vi "Process.vi"(8 "error in":errorcluster, 11 "Inst.RP100":refnum<class "Inst.RP100.lvclass">) -> (0 "error out":errorcluster, 3 "Inst.RP100 out":refnum<class "Inst.RP100.lvclass">)   [LabVIEW 2019, in "Inst.RP100.lvlib" / "Inst.RP100.lvclass"]
doc: "---------------------------------------------------------------\nJKI State Machine Objects™\nhttp://jki.net/state-machine-objects/\nCopyright (C) 2005-2015, JKI <info@jki.net>\nALL RIGHTS RESERVED"
uses:
  Inst.RP100.lvclass
  C:/Program Files (x86)/National Instruments/LabVIEW 2019/vi.lib/JKI/JKI SMO/SMO/SMO.lvclass
  C:/Program Files (x86)/National Instruments/LabVIEW 2019/user.lib/LevyLab/Instrument Framework/Instrument/Instrument.lvclass
  Typedefs/PrivateEvents--Inst.RP100.MessageToProcess.ctl
  <userlib>/LevyLab/RemoteControl/RemoteControl/Typedefs/Message--Cluster.ctl
  <vilib>/JKI/JKI SMO/SMO/SMO.lvclass/SMO.ctl
  Inst.RP100.lvclass/Inst.RP100.ctl
  <vilib>/JKI/JKI SMO/SMO/Private/ReftoDVR--SMO.vi
  <userlib>/LevyLab/Instrument Framework/Instrument Types/Strain/Instrument.Strain.lvclass
  <vilib>/JKI/JKI SMO/SMO/SMO.lvclass
  <userlib>/LevyLab/Instrument Framework/Instrument/Instrument.lvclass
  <userlib>/LevyLab/RemoteControl/RemoteControl/RemoteControl.lvclass
  <userlib>/LevyLab/Debug/Debug.lvlib
panel:
  out "Status":string
  out "State History":string
  # "Inst.RP100"
  # "Inst.RP100"
  # "For instructions on how to use the JKI State Machine Objects, examples and video tutorials, visit:\nhttp://jki.net/state-machine-objects/\n\nJKI State Machine Objects™\nhttp://jki.net/state-machine-objects/\nCopyright (C) 2005-2015, JKI <info@jki.net>\nALL RIGHTS RESERVED"
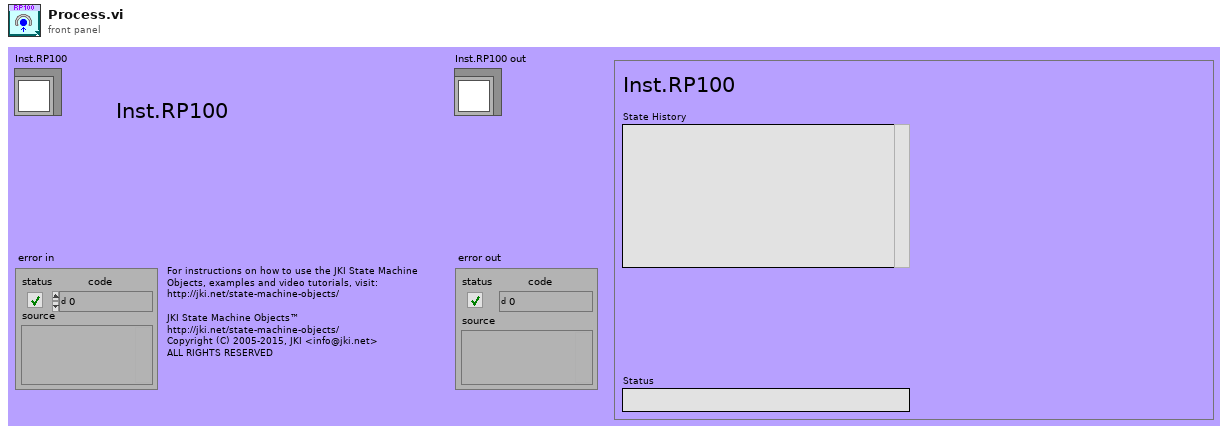
[diagram p1: front panel]
types:
  T1 = enum32{"invalid app kind", "Development System", "Run Time System", "Student Edition", "Embedded LabVIEW", "Evaluation", "Custom"}
  T2 = enum32{"Invalid", "Standard", "Closed", "Hidden", "Minimized", "Maximized"}
  T3 = typedef "RemoteControl.lvclass/Message--Cluster.ctl" = cluster{"Command":string, "Data":variant, "ID":string}
  T4 = typedef "Inst.RP100.lvlib/Inst.RP100.lvclass/PrivateEvents--Inst.RP100.MessageToProcess.ctl" = cluster{"Message":T5}
  T5 = typedef "RemoteControl.lvlib/RemoteControl.lvclass/Message--Cluster.ctl" = cluster{"Command":string, "Data":variant, "ID":string}
  T6 = cluster{"Core":cluster{"Current VI Reference":refnum<vi>, "Close Panel on Exit?":bool, "Last Error":cluster{"error":errorcluster, "previous state":string, "remaining states":string}, "Shutdown?":bool}, "SelfRef":refnum<class "Inst.RP100.lvclass">, "Running Step":i32, "sequence":string[], "MessageToProcess":T4}
  T7 = cluster{"Current VI Reference":refnum<vi>, "Close Panel on Exit?":bool, "Last Error":cluster{"error":errorcluster, "previous state":string, "remaining states":string}, "Shutdown?":bool}
  T8 = typedef "Debug.lvlib/Attribute.Debug.lvclass/DebugBehavior.ctl" = enum16{"Normal", "Debug"}
  T9 = typedef "smo.lvlib/SMO.lvclass/Protected Events.ctl" = cluster{"StopProcesses":refnum<user-event>, "AbortProcesses":refnum<user-event>, "Config Changed":refnum<user-event>, "Dependency":refnum<user-event>}
  T10 = typedef "Inst.RP100.lvlib/Inst.RP100.lvclass/Inst.RP100.getAll--Cluster.ctl" = cluster{"OutputStateCh1":string, "OutputStateCh2":string, "LevelCh1":dbl, "LevelCh2":dbl, "SlewCh1":dbl, "SlewCh2":dbl, "MeasuredVCh1":dbl, "MeasuredVCh2":dbl, "MeasuredICh1":dbl, "MeasuredICh2":dbl}
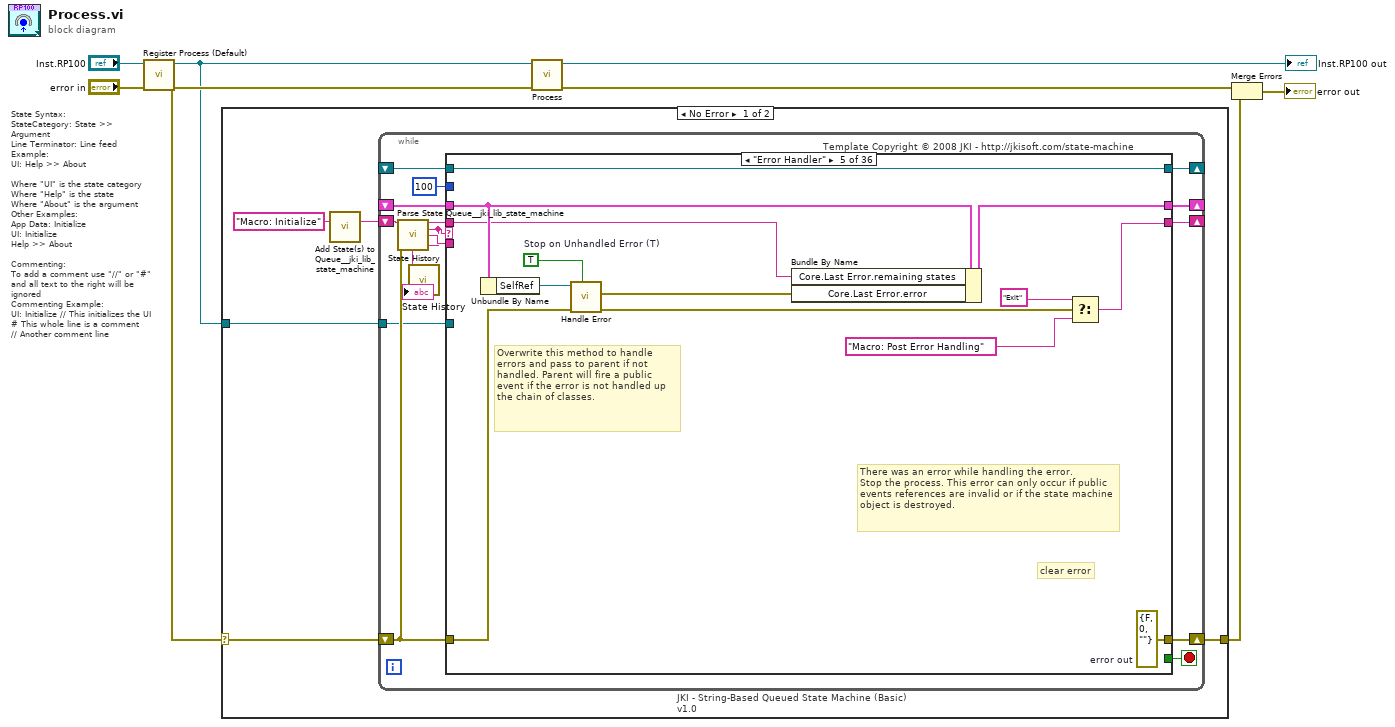
[diagram p0: block diagram]
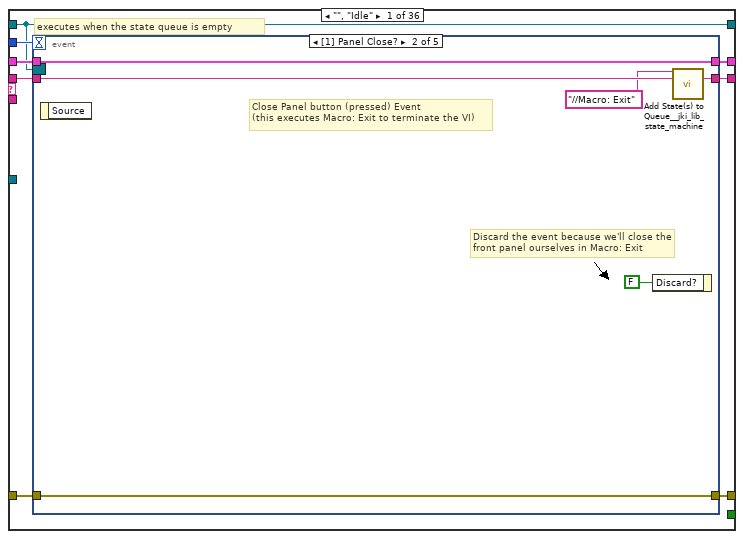
[diagram p2: hidden frame]
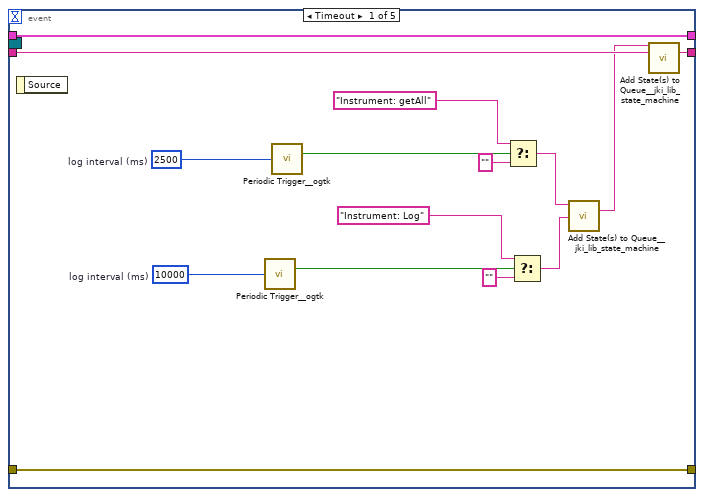
[diagram p3: hidden frame]
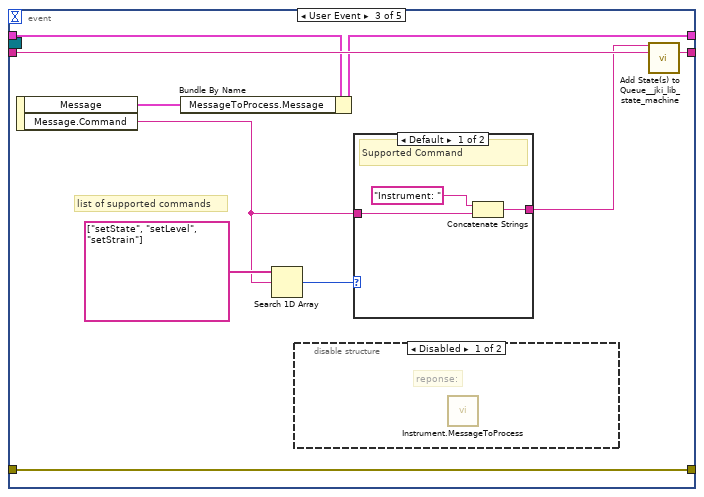
[diagram p4: hidden frame]
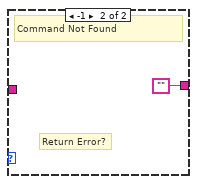
[diagram p6: hidden frame]
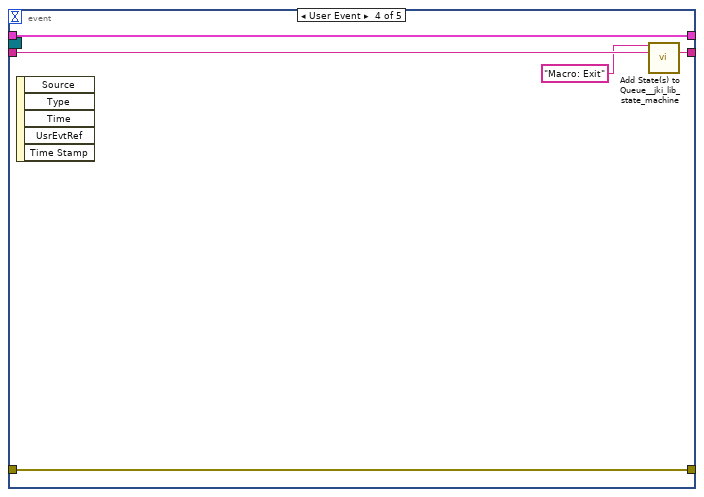
[diagram p7: hidden frame]
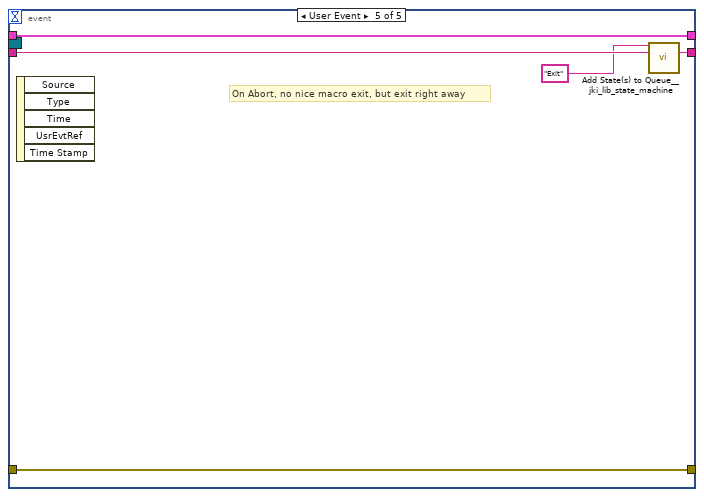
[diagram p8: hidden frame]
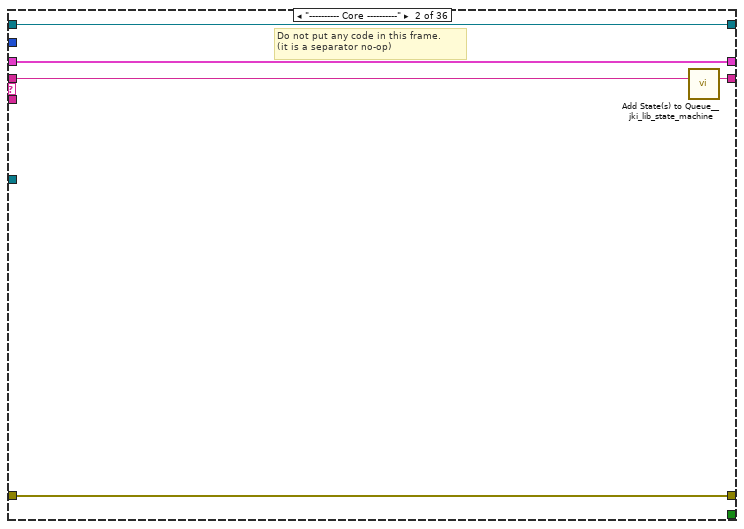
[diagram p9: hidden frame]
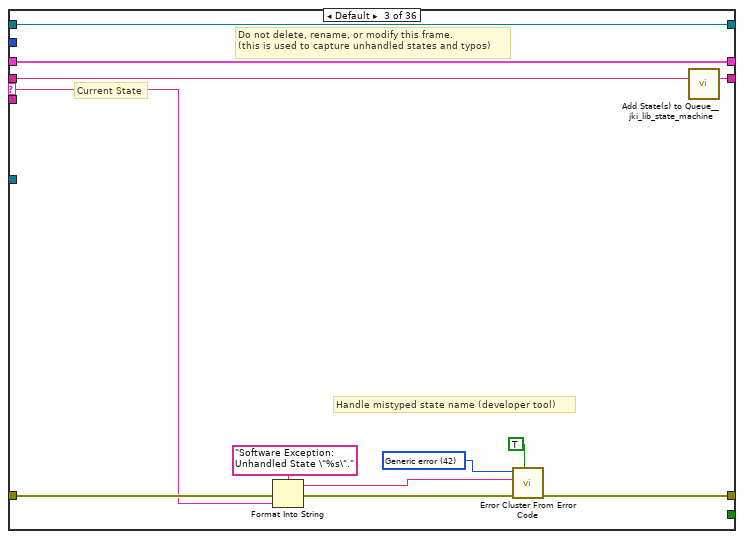
[diagram p10: hidden frame]
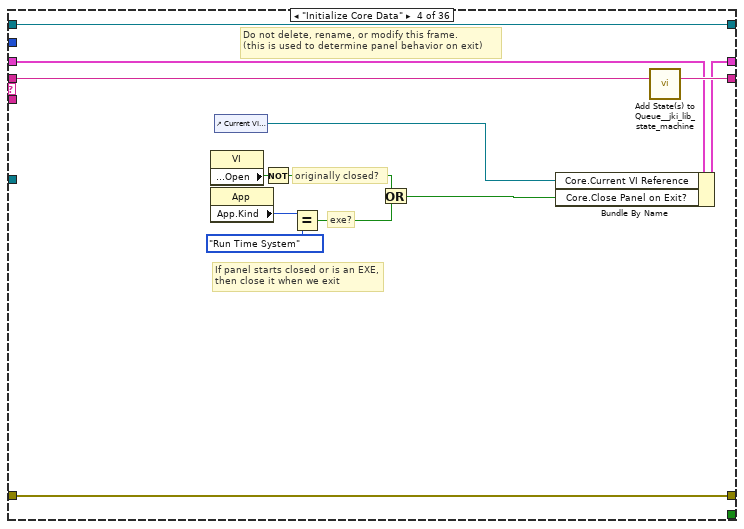
[diagram p11: hidden frame]
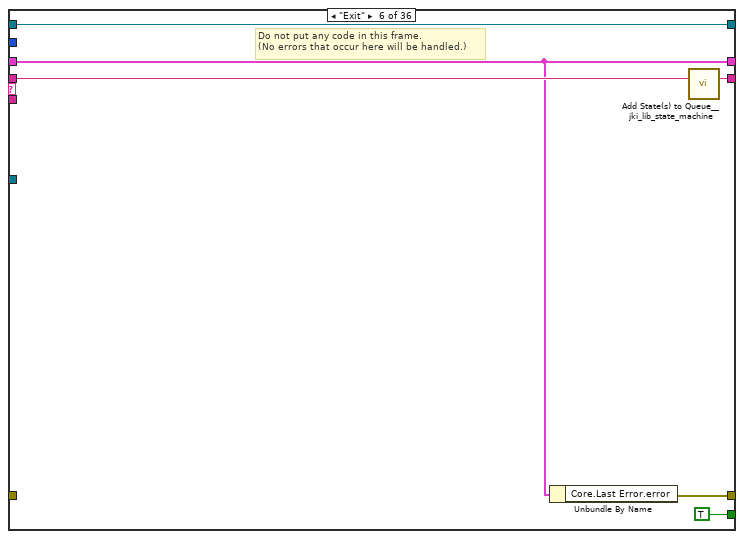
[diagram p12: hidden frame]
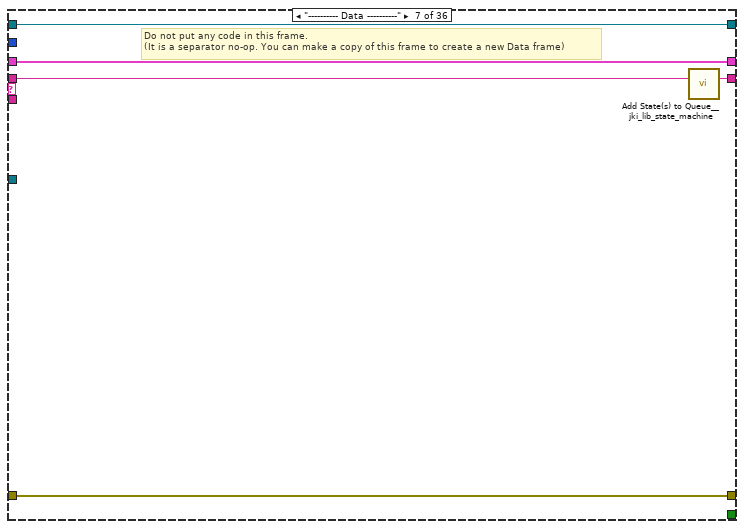
[diagram p13: hidden frame]
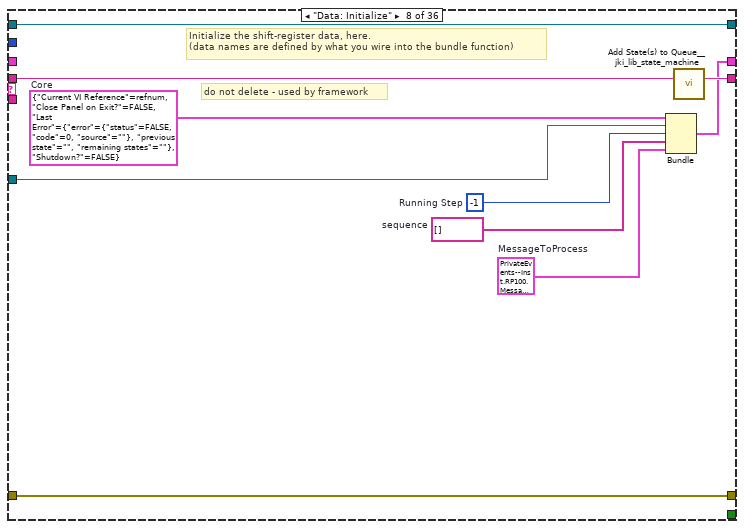
[diagram p14: hidden frame]
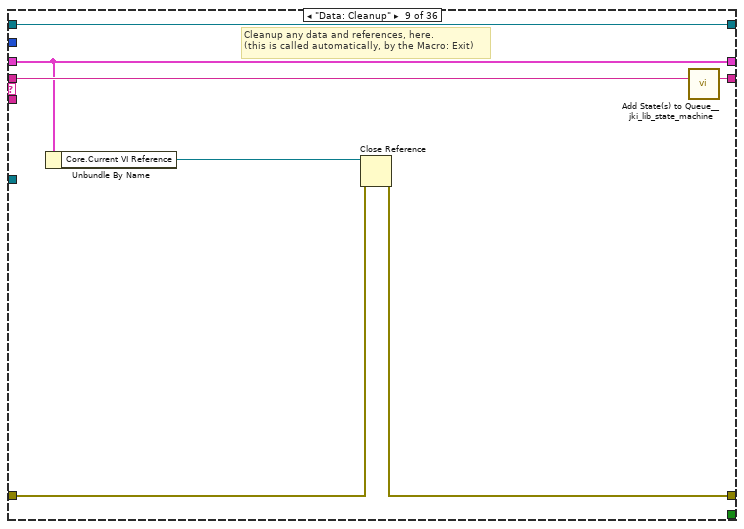
[diagram p15: hidden frame]
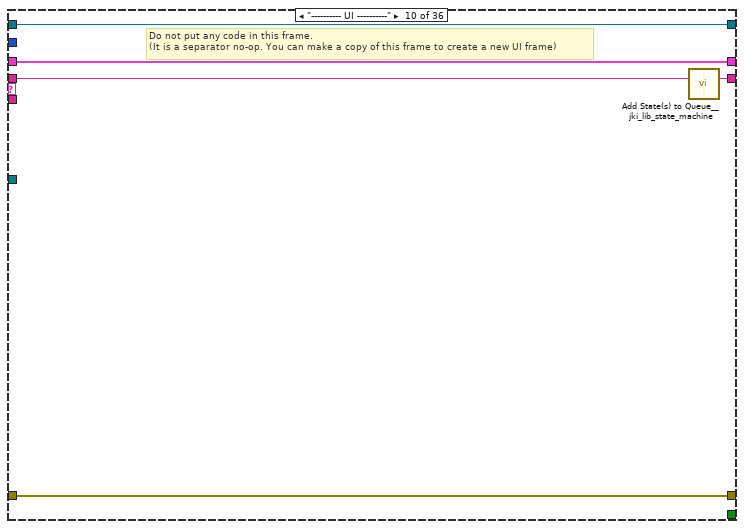
[diagram p16: hidden frame]
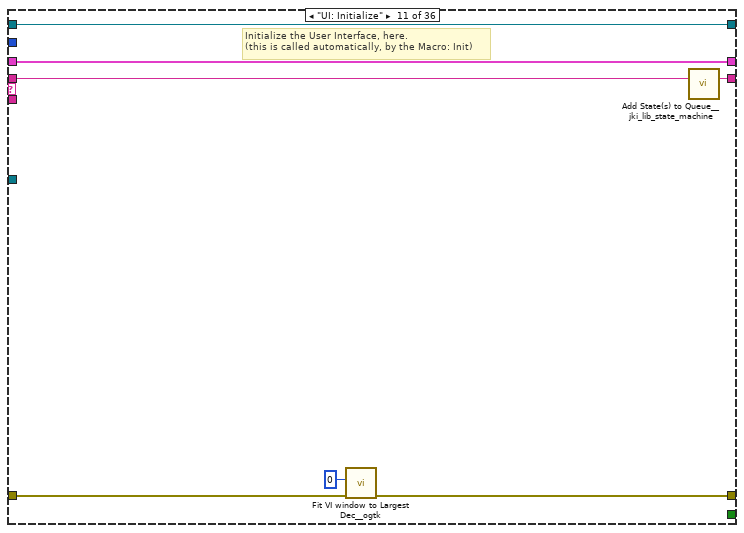
[diagram p17: hidden frame]
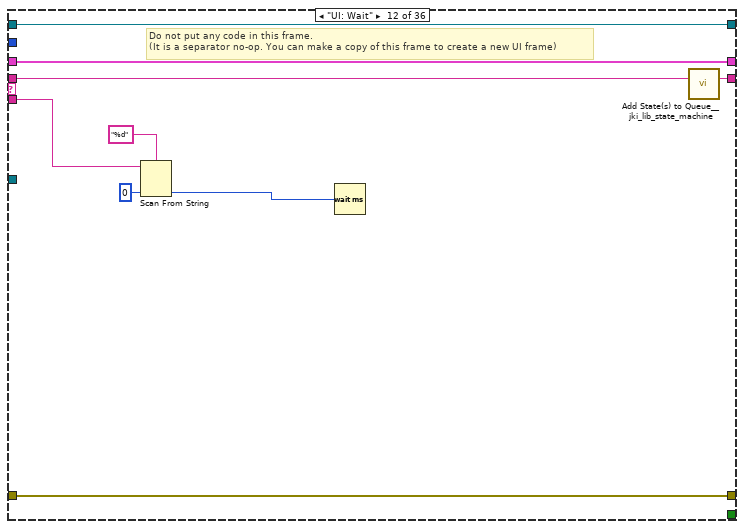
[diagram p18: hidden frame]
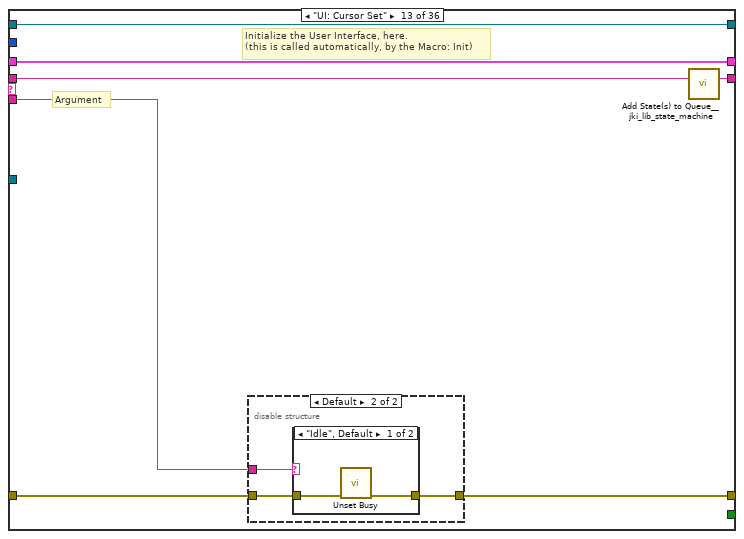
[diagram p19: hidden frame]
diagram:
  # "State Syntax:\nStateCategory: State >> Argument\nLine Terminator: Line feed\nExample:\nUI: Help >> About\n\nWhere \"UI\" is the state category\nWhere \"Help\" is the state\nWhere \"About\" is the argument\nOther Examples:\nApp Data: Initialize\nUI: Initialize\nHelp >> About\n\nCommenting:\nTo add a comment use \"//\" or \"#\" and all text to the right will be ignored\nCommenting Example:\nUI: Initialize // This initializes the UI\n# This whole line is a comment\n// Another comment line"
  n1 = call <vilib>:"Register Process (Default).vi"("error in (no error)"="error in", "SMO"="Inst.RP100") -> ("error out"=w5:errorcluster, "SelfRef"=w4:refnum<class "Inst.RP100.lvclass">)  [unwired: 8 in]
  n2 = case shown="No Error" w5 {
    selector: w5 -> [w10 w458]
    tunnel: w4 -> [w11 _]
    tunnel: [w9 w458] -> w1
    frame No Error {
      n3 = call <vilib>:"Add State(s) to Queue__jki_lib_state_machine.vi"("State(s) in (\"\")"="Macro: Initialize") -> ("States Out"=w13:string)  [unwired: 14 in]
      n4 = while "JKI - String-Based Queued State Machine (Basic) v1.0" {
        shift-right: [w22] -> _
        shift-left: _ -> [w21]
        shift-right: [w25] -> w9
        shift-left: w10 -> [w19]
        shift-right: [w24] -> _
        shift-left: w13 -> [w26]
        tunnel: w11 -> [w18]
        shift-right: [w17] -> _
        shift-left: _ -> [w16]
        stop <- w23 stop-if-true
        # "Template Copyright © 2008 JKI - http://jkisoft.com/state-machine"
        n5 = call <vilib>:"Parse State Queue__jki_lib_state_machine.vi"("State Queue"=w26, "Error In (no error)"=w19) -> ("Remaining States"=w28:string, "Current State"=w15:string, "Arguments"=w27:string)  [unwired: 11 in]
        n6 = call <userlib>:"State History.vi"("Current State"=w15) -> ("History"=→"State History":string)  [unwired: 10 in]
        n7 = case shown="\"Error Handler\"" w15 {
          selector: w15 -> [_ _ w88 _ _ _ _ _ _ _ _ _ _ _ _ _ _ _ _ _ _ _ _ _ _ _ _ _ _ _ _ _ _ _ _ _]
          tunnel: w28 -> [w36 w86 w92 w111 w116 w130 w135 w145 w152 w157 w164 w173 w180 w196 w228 w237 w252 w269 w290 w307 w312 w323 w328 w341 w347 w354 w363 w372 w382 w392 w402 w414 w427 w432 w438 w457]
          tunnel: w27 -> [_ _ _ _ _ _ _ _ _ _ _ w165 w174 w190 _ _ _ _ _ _ _ _ _ _ _ _ _ _ _ _ _ _ _ _ w433 w441]
          tunnel: w21 -> [w34 w83 w90 w102 w120 w126 w132 _ w146 w154 w162 w170 w178 w192 w225 w234 w241 w259 w280 w291 w309 w320 w325 w334 w345 w349 w359 w368 w378 w388 w398 w410 w423 w428 w434 w447]
          tunnel: [w33 w84 w94 w108 w121 w125 w133 w137 w148 w155 w159 w171 w175 w193 w226 w229 w239 w267 w288 w294 w310 w314 w326 w337 w343 w351 w356 w365 w374 w384 w394 w403 w417 w429 w435 w449] -> w25
          tunnel: w19 -> [w32 w84 w93 w108 w122 _ w133 w137 w149 w155 w158 w171 w176 w194 w226 w229 w238 w267 w288 w294 w310 w315 w326 w331 w343 w351 w355 w364 w375 w385 w395 w408 w418 w429 w435 w443]
          tunnel: [w35 w85 w91 w110 w112 w129 w134 w144 w151 w156 w163 w172 w179 w195 w227 w236 w251 w268 w289 w306 w311 w322 w327 w340 w346 w353 w362 w371 w381 w391 w401 w413 w426 w431 w437 w456] -> w24
          tunnel: [_ _ _ _ _ TRUE _ _ _ _ _ _ _ _ _ _ _ _ _ _ _ _ _ _ _ _ _ _ _ _ _ _ _ _ _ _] -> w23
          tunnel: [w31 w83 w90 w109 w119 w126 w132 w143 w146 w154 w162 w170 w178 w192 w225 w234 w242 w260 w281 w292 w309 w320 w325 w334 w345 w350 w360 w369 w379 w389 w399 w411 w424 w428 w434 w446] -> w22
          tunnel: 100 ("Timeout") -> [w30 _ _ _ _ _ _ _ _ _ _ _ _ _ _ _ _ _ _ _ _ _ _ _ _ _ _ _ _ _ _ _ _ _ _ _]
          tunnel: w18 -> [_ _ _ _ _ _ _ w138 _ _ _ _ _ _ _ _ _ _ _ _ _ _ _ _ _ _ _ _ _ _ _ _ _ _ _ _]
          tunnel: [w29 w82 w87 w99 w124 w127 w131 w142 w147 w153 w161 w169 w177 w189 w224 w235 w250 w266 w287 w301 w308 w321 w324 w339 w344 w352 w361 w370 w380 w390 w400 w412 w425 w430 w436 w455] -> w17
          tunnel: w16 -> [w29 w82 w87 w99 w124 w127 w131 w142 w147 w153 w161 w169 w177 w189 w224 w235 w250 w266 w287 w301 w308 w321 w324 _ w344 w352 w361 w370 w380 w390 w400 w412 w425 w430 w436 w455]
          frame "", "Idle" {
            # "executes when the state queue is empty"
            n8 = event shown="[1] Panel Close?" {
              selector: w29 -> [_ _ _ _ _]
              dyn-events: _ -> [_ _ _ _ _]
              timeout: w30 -> [_ _ _ _ _]
              tunnel: w36 -> [w51 w57 w67 w76 w81]
              tunnel: [w50 w56 w66 w75 w80] -> w35
              tunnel: w34 -> [w48 w54 w59 w73 w78]
              tunnel: [w49 w55 w65 w74 w79] -> w33
              tunnel: w32 -> [w49 w55 w65 w74 w79]
              tunnel: [w48 w54 w60 w73 w78] -> w31
              event Timeout {
                w41 = u32 10000  # log interval (ms)
                w45 = u32 2500  # log interval (ms)
                n9 = event-data() -> ()  [unwired: 1 in, 1 out]
                n10 = call <userlib>:"Periodic Trigger__ogtk.vi"("time (ms)"=w41) -> ("Triggered"=w40:bool)  [unwired: 12 in, 2 out]
                n11 = call <userlib>:"Periodic Trigger__ogtk.vi"("time (ms)"=w45) -> ("Triggered"=w47:bool)  [unwired: 12 in, 2 out]
                n12 = Select(t="Instrument: getAll", s=w47, f="") -> (s? t:f=w38:string)
                n13 = Select(t="Instrument: Log", s=w40, f="") -> (s? t:f=w39:string)
                n14 = call <vilib>:"Add State(s) to Queue__jki_lib_state_machine.vi"("State(s) in Front (\"\")"=w38, "State(s) at Back (\"\")"=w39) -> ("States Out"=w37:string)  [unwired: 13 in]
                n15 = call <vilib>:"Add State(s) to Queue__jki_lib_state_machine.vi"("State(s) in Front (\"\")"=w37, "State(s) in (\"\")"=w51) -> ("States Out"=w50:string)  [unwired: 13 in]
              }
              event Panel Close? {
                # "Discard the event because we'll close the front panel ourselves in Macro: Exit"
                # "Close Panel button (pressed) Event\n(this executes Macro: Exit to terminate the VI)"
                n16 = event-data() -> ()  [unwired: 1 in, 1 out]
                n17 = event-data("Discard?"=FALSE) -> ()  [unwired: 1 in, 1 out]
                n18 = call <vilib>:"Add State(s) to Queue__jki_lib_state_machine.vi"("State(s) in Front (\"\")"="//Macro: Exit", "State(s) in (\"\")"=w57) -> ("States Out"=w56:string)  [unwired: 13 in]
              }
              event User Event {
                # "list of supported commands"
                n19 = event-data() -> ("Message"=w58:T3, "Message.Command"=w61:string)  [unwired: 1 in]
                n20 = Bundle By Name(cluster=w59, "MessageToProcess.Message"=w58) -> (w60:T6)
                n21 = Search 1D Array(1D array=string[] ["setState", "setLevel", "setStrain"], element=w61) -> (index of element=w64:i32)  [unwired: 1 in]
                n22 = disable-structure shown="Disabled" {
                  frame Disabled {
                    # "reponse:"
                    n23 = call <userlib>:"Instrument.MessageToProcess.vi"() -> ()  [unwired: 10 in, 2 out]
                  }
                  frame Enabled {
                  }
                }
                n24 = case shown="Default" w64 {
                  tunnel: [w70 "" ("Empty String Constant")] -> w62
                  tunnel: w61 -> [w69 _]
                  frame Default {
                    # "Supported Command"
                    n25 = Concatenate Strings("Instrument: ", w69) -> (w70:string)
                  }
                  frame -1 {
                    # "Return Error?"
                    # "Command Not Found"
                  }
                }
                n26 = call <vilib>:"Add State(s) to Queue__jki_lib_state_machine.vi"("State(s) in Front (\"\")"=w62, "State(s) in (\"\")"=w67) -> ("States Out"=w66:string)  [unwired: 13 in]
              }
              event User Event {
                n27 = event-data() -> ()  [unwired: 1 in, 5 out]
                n28 = call <vilib>:"Add State(s) to Queue__jki_lib_state_machine.vi"("State(s) in Front (\"\")"="Macro: Exit", "State(s) in (\"\")"=w76) -> ("States Out"=w75:string)  [unwired: 13 in]
              }
              event User Event {
                # "On Abort, no nice macro exit, but exit right away"
                n29 = event-data() -> ()  [unwired: 1 in, 5 out]
                n30 = call <vilib>:"Add State(s) to Queue__jki_lib_state_machine.vi"("State(s) in Front (\"\")"="Exit", "State(s) in (\"\")"=w81) -> ("States Out"=w80:string)  [unwired: 13 in]
              }
            }
          }
          frame "---------- Core ----------" {
            # "Do not put any code in this frame.\n(it is a separator no-op)"
            n31 = call <vilib>:"Add State(s) to Queue__jki_lib_state_machine.vi"("State(s) in (\"\")"=w86) -> ("States Out"=w85:string)  [unwired: 14 in]
          }
          frame Default {
            w97 = 42 items=["No error", "Argument error", "Memory is full", "Out of zone", "End of file", "File already open", "Generic file I/O error", "File not found", "File permission error", "Disk is full", "Duplicate path", "Too many files open", "System feature not enabled", "Resource file not found", "Cannot add resource", "Resource not found", "Image not found", "Image memory error", "Pen does not exist", "Config type invalid", "Config token not found", "Config parse error", "Config memory error", "Bad external code format", "Bad external code offset", "External code not present", "Null window", "Destroy window error", "Null menu", "Print aborted", "Bad print record", "Print driver error", "Windows error during printing", "Memory error during printing", "Print dialog error", "Generic print error", "Invalid device refnum", "Device not found", "Device parameter error", "Device unit error", "Cannot open device", "Device call aborted", "Generic error", "Cancelled by user", "Object ID too low", "Object ID too high", "Object not in heap", "Unknown heap", "Unknown object (invalid DefProc)", "Unknown object (DefProc not in table)", "Message out of range", "Invalid (null) method", "Unknown message", "Manager call not supported", "Bad address", "Network operation in progress", "Network operation timed out", "Connection is busy", "Network attribute not supported", "Network error", "Address in use", "System out of memory", "Connection aborted", "Connection refused", "Not connected", "Already connected", "Connection closed", "Initialization error (interapplication manager)", "Bad occurrence", "Wait on unbound occurrence handler", "Occurrence queue overflow", "Datalog type conflict", "Unused", "Unrecognized type (interapplication manager)", "Memory corrupt", "Failed to make temporary DLL", "Old CIN version", "Drag socket not found", "Failed to load drop-object", "Failed to register OLE object", "Failed to release OLE object", "Format specifier type mismatch", "Unknown format specifier", "Too few format specifiers", "Too many format specifiers", "Scan failed", "Newer CIN version", "Error converting to variant", "Runtime menu error", "Password tampered", "Variant attribute not found", "Incompatible variant data type", "Event data is not available", "Event Store is not present", "Occurrence is not found", "Event Queue is not created", "Event info is not available", "Refnum passed is NULL", "Error retrieving Class GUID", "Error retrieving CoClass GUID", "Error retrieving TypeLib GUID.", "Bad built application magic bytes.", "Specific driver is different from the specific driver associated with the Logical Name.", "There is no session opened to the class driver.", "Max Error", "MAX - Error with config objects", "MAX - Error loading configuration", "MAX - Group not supported"]
            # "Current State"
            # "Do not delete, rename, or modify this frame.\n(this is used to capture unhandled states and typos)"
            # "Handle mistyped state name (developer tool)"
            n32 = Format Into String(format string="Software Exception: Unhandled State \"%s\"." ("message"), error in=w93, w88) -> (resulting string=w96:string, error out=w95:errorcluster)  [unwired: 1 in]
            n33 = call <vilib>:"Error Cluster From Error Code.vi"("show call chain? (False)"=TRUE, "error in (no error)"=w95, "error message (\"\")"=w96, "error code (0)"=w97) -> ("error out"=w94:errorcluster)  [unwired: 5 in]
            n34 = call <vilib>:"Add State(s) to Queue__jki_lib_state_machine.vi"("State(s) in (\"\")"=w92) -> ("States Out"=w91:string)  [unwired: 14 in]
          }
          frame "Initialize Core Data" {
            # "Do not delete, rename, or modify this frame.\n(this is used to determine panel behavior on exit)"
            # "originally closed?"
            # "exe?"
            # "If panel starts closed or is an EXE, then close it when we exit"
            n35 = property class="VI"() -> ("Front Panel.Open"=w107:bool)  [unwired: 2 in, 2 out]
            n36 = property class="App"() -> ("App.Kind"=w106:T1)  [unwired: 2 in, 2 out]
            n37 = control-ref of="Current VI Reference"() -> (w100:refnum<vi>)
            n38 = Not(x=w107) -> (.not. x?=w104:bool)
            n39 = Equal?(x=w106, y=T1."Run Time System" ("Application:Kind")) -> (x = y?=w103:bool)
            n40 = Or(x=w104, y=w103) -> (x .or. y?=w101:bool)
            n41 = Bundle By Name(cluster=w102, "Core.Current VI Reference"=w100, "Core.Close Panel on Exit?"=w101) -> (w109:T6)
            n42 = call <vilib>:"Add State(s) to Queue__jki_lib_state_machine.vi"("State(s) in (\"\")"=w111) -> ("States Out"=w110:string)  [unwired: 14 in]
          }
          frame "Error Handler" {
            w117 = TRUE  # Stop on Unhandled Error (T)
            w121 = errorcluster {"status"=FALSE, "code"=0, "source"=""}  # error out
            # "clear error"
            # "There was an error while handling the error.\nStop the process. This error can only occur if public events references are invalid or if the state machine object is destroyed."
            # "Overwrite this method to handle errors and pass to parent if not handled. Parent will fire a public event if the error is not handled up the chain of classes."
            n43 = Unbundle By Name(w120) -> ("SelfRef"=w123:refnum<class "Inst.RP100.lvclass">)
            n44 = call-dynamic "Handle Error.vi"("Stop on Unhandled Error (T)"=w117, "error in"=w122, "SMO"=w123) -> ("handling error"=w113:errorcluster, "Unhandled error"=w118:errorcluster)  [unwired: 6 in, 1 out]
            n45 = Bundle By Name(cluster=w120, "Core.Last Error.remaining states"=w116, "Core.Last Error.error"=w118) -> (w119:T6)
            n46 = Select(t="Exit", s=w113, f="Macro: Post Error Handling") -> (s? t:f=w112:string)
          }
          frame "Exit" {
            # "Do not put any code in this frame.\n(No errors that occur here will be handled.)"
            n47 = Unbundle By Name(w126) -> ("Core.Last Error.error"=w125:errorcluster)
            n48 = call <vilib>:"Add State(s) to Queue__jki_lib_state_machine.vi"("State(s) in (\"\")"=w130) -> ("States Out"=w129:string)  [unwired: 14 in]
          }
          frame "---------- Data ----------" {
            # "Do not put any code in this frame.\n(It is a separator no-op. You can make a copy of this frame to create a new Data frame)"
            n49 = call <vilib>:"Add State(s) to Queue__jki_lib_state_machine.vi"("State(s) in (\"\")"=w135) -> ("States Out"=w134:string)  [unwired: 14 in]
          }
          frame "Data: Initialize" {
            w136 = T4 {"Message"={"Command"="", "Data"=variant(string ""), "ID"=""}}  # MessageToProcess
            w139 = string[] []  # sequence
            w140 = -1  # Running Step
            w141 = T7 {"Current VI Reference"=refnum, "Close Panel on Exit?"=FALSE, "Last Error"={"error"={"status"=FALSE, "code"=0, "source"=""}, "previous state"="", "remaining states"=""}, "Shutdown?"=FALSE}  # Core
            # "do not delete - used by framework"
            # "Initialize the shift-register data, here.\n(data names are defined by what you wire into the bundle function)"
            n50 = Bundle("Core"=w141, "SelfRef"=w138, "Running Step"=w140, "sequence"=w139, "MessageToProcess"=w136) -> (w143:T6)  [unwired: 1 in]
            n51 = call <vilib>:"Add State(s) to Queue__jki_lib_state_machine.vi"("State(s) in (\"\")"=w145) -> ("States Out"=w144:string)  [unwired: 14 in]
          }
          frame "Data: Cleanup" {
            # "Cleanup any data and references, here.\n(this is called automatically, by the Macro: Exit)"
            n52 = Unbundle By Name(w146) -> ("Core.Current VI Reference"=w150:refnum<vi>)
            n53 = Close Reference(reference=w150, error in (no error)=w149) -> (error out=w148:errorcluster)
            n54 = call <vilib>:"Add State(s) to Queue__jki_lib_state_machine.vi"("State(s) in (\"\")"=w152) -> ("States Out"=w151:string)  [unwired: 14 in]
          }
          frame "---------- UI ----------" {
            # "Do not put any code in this frame.\n(It is a separator no-op. You can make a copy of this frame to create a new UI frame)"
            n55 = call <vilib>:"Add State(s) to Queue__jki_lib_state_machine.vi"("State(s) in (\"\")"=w157) -> ("States Out"=w156:string)  [unwired: 14 in]
          }
          frame "UI: Initialize" {
            # "Initialize the User Interface, here.\n(this is called automatically, by the Macro: Init)"
            n56 = call <userlib>:"Fit VI window to Largest Dec__ogtk.vi"("error in (no error)"=w158, "border spacing (2 px)"=0) -> ("error out"=w159:errorcluster)  [unwired: 4 in, 1 out]
            n57 = call <vilib>:"Add State(s) to Queue__jki_lib_state_machine.vi"("State(s) in (\"\")"=w164) -> ("States Out"=w163:string)  [unwired: 14 in]
          }
          frame "UI: Wait" {
            # "Do not put any code in this frame.\n(It is a separator no-op. You can make a copy of this frame to create a new UI frame)"
            n58 = Scan From String(format string="%d", input string=w165, default 1=u32 0 ("default value 1")) -> (output 1=w166:u32)  [unwired: 2 in, 3 out]
            n59 = Wait (ms)(milliseconds to wait=w166) -> ()  [unwired: 1 out]
            n60 = call <vilib>:"Add State(s) to Queue__jki_lib_state_machine.vi"("State(s) in (\"\")"=w173) -> ("States Out"=w172:string)  [unwired: 14 in]
          }
          frame "UI: Cursor Set" {
            # "Argument"
            # "Initialize the User Interface, here.\n(this is called automatically, by the Macro: Init)"
            n61 = disable-structure shown="Default" {
              disable-tunnel: w176 -> [w181 w184]
              disable-tunnel: [w181 w183] -> w175
              disable-tunnel: w174 -> [_ w182]
              frame condition #0 {
              }
              frame condition #1 (active) {
                n62 = case shown="\"Idle\", Default" w182 {
                  tunnel: w184 -> [w186 w188]
                  tunnel: [w185 w187] -> w183
                  frame "Idle", Default {
                    n63 = call <vilib>:"Unset Busy.vi"("error in (no error)"=w186) -> ("error out"=w185:errorcluster)  [unwired: 10 in]
                  }
                  frame "Busy" {
                    n64 = call <vilib>:"Set Busy.vi"("error in (no error)"=w188) -> ("error out"=w187:errorcluster)  [unwired: 9 in, 1 out]
                  }
                }
              }
            }
            n65 = call <vilib>:"Add State(s) to Queue__jki_lib_state_machine.vi"("State(s) in (\"\")"=w180) -> ("States Out"=w179:string)  [unwired: 14 in]
          }
          frame "UI: Front Panel State" {
            # "Argument"
            # "Set Front Panel Open or Closed\n(Usage: \"UI: Front Panel State >> Open|Close\")"
            n66 = Unbundle By Name(w192) -> ("Core.Current VI Reference"=w191:refnum<vi>)
            n67 = disable-structure shown="Default" {
              disable-tunnel: w194 -> [w200 w223]
              disable-tunnel: [w199 w223] -> w193
              disable-tunnel: w191 -> [w198 _]
              disable-tunnel: w190 -> [w197 _]
              frame condition #0 (active) {
                n68 = case shown="\"Close\"" w197 {
                  tunnel: w200 -> [w204 w217]
                  tunnel: [w206 w218] -> w199
                  tunnel: w198 -> [w205 w215]
                  frame "Open", Default {
                    n69 = property class="VI"(reference=w205, error in=w204) -> (reference out=w202:refnum<vi>, error out=w203:errorcluster, "FP.State"=w201:T2)
                    n70 = case shown="\"Closed\"" w201 {
                      tunnel: [w209 w212] -> w206
                      tunnel: w203 -> [w208 w212]
                      tunnel: w202 -> [w207 _]
                      frame "Closed" {
                        n71 = invoke class="VI" method="FP.Open"(reference=w207, error in=w208, "Activate"=TRUE, "State"=T2."Standard") -> (error out=w209:errorcluster)  [unwired: 1 in, 4 out]
                      }
                      frame Default {
                      }
                    }
                  }
                  frame "Close" {
                    n72 = property class="VI"(reference=w215, error in=w217) -> (reference out=w214:refnum<vi>, error out=w216:errorcluster, "FP.State"=w213:T2)
                    n73 = case shown="Default" w213 {
                      tunnel: [w219 w222] -> w218
                      tunnel: w216 -> [w219 w221]
                      tunnel: w214 -> [_ w220]
                      frame "Invalid", "Closed" {
                      }
                      frame Default {
                        n74 = invoke class="VI" method="FP.Close"(reference=w220, error in=w221) -> (error out=w222:errorcluster)  [unwired: 1 in, 2 out]
                      }
                    }
                  }
                }
              }
              frame condition #1 {
              }
            }
            n75 = call <vilib>:"Add State(s) to Queue__jki_lib_state_machine.vi"("State(s) in (\"\")"=w196) -> ("States Out"=w195:string)  [unwired: 14 in]
          }
          frame "---------- Macro ----------" {
            # "Do not put any code in this frame.\n(It is a separator no-op. You can make a copy of this frame to create a new Macro frame)"
            n76 = call <vilib>:"Add State(s) to Queue__jki_lib_state_machine.vi"("State(s) in (\"\")"=w228) -> ("States Out"=w227:string)  [unwired: 14 in]
          }
          frame "Macro: Initialize" {
            # "Initialization Macro\n(This is called once, when the VI starts)"
            n77 = call <vilib>:"Add State(s) to Queue__jki_lib_state_machine.vi"("State(s) in Front (\"\")"="Data: Initialize\nInitialize Core Data\nEvents: Register", "State(s) in (\"\")"="Process: Sync", "State(s) at Back (\"\")"="UI: Initialize\nUI: Front Panel State >> Close\nInstrument: Open Hardware\nMacro: Debug") -> ("States Out"=w232:string)  [unwired: 12 in]
            n78 = call <vilib>:"Add State(s) to Queue__jki_lib_state_machine.vi"("State(s) in Front (\"\")"=w232, "State(s) in (\"\")"=w237) -> ("States Out"=w236:string)  [unwired: 13 in]
          }
          frame "Macro: Debug" {
            # "exe?"
            # "If pane is an EXE, then close it when we exit"
            # "Macro: Debug\n(get debug behavior, determine UI and determine shutdown behavior)"
            n79 = Unbundle By Name(w241) -> ("Core.Close Panel on Exit?"=w244:bool, "SelfRef"=w249:refnum<class "Inst.RP100.lvclass">)
            n80 = property class="App"() -> ("App.Kind"=w247:T1)  [unwired: 2 in, 2 out]
            n81 = Equal?(x=w247, y=T1."Run Time System" ("Application:Kind")) -> (x = y?=w243:bool)
            n82 = call <userlib>:"Get Debug Mode.vi"("error in (no error)"=w238, "SMO"=w249) -> ("error out"=w239:errorcluster, "Behavior"=w248:T8)  [unwired: 7 in, 1 out]
            n83 = case shown="\"Debug\"" w248 {
              tunnel: [w253 w255] -> w245
              tunnel: w244 -> [w253 _]
              tunnel: w243 -> [_ w257]
              tunnel: [_ "UI: Front Panel State >> Open\nUI: Wait >> 1000"] -> w240
              frame "Normal", Default {
                # "respect core.close"
              }
              frame "Debug" {
                # "keep panel open\nunless exe"
                n84 = Or(x=w257, y=FALSE) -> (x .or. y?=w255:bool)
              }
            }
            n85 = Bundle By Name(cluster=w241, "Core.Close Panel on Exit?"=w245) -> (w242:T6)
            n86 = call <vilib>:"Add State(s) to Queue__jki_lib_state_machine.vi"("State(s) in Front (\"\")"=w240, "State(s) in (\"\")"=w252) -> ("States Out"=w251:string)  [unwired: 13 in]
          }
          frame "Macro: Post Error Handling" {
            # "Clear Last Error?"
            n87 = Unbundle By Name(w259) -> ("Core.Last Error.remaining states"=w261:string, "Core.Shutdown?"=w262:bool)
            n88 = Unbundle By Name(w259) -> ("Core.Last Error.error"=w265:errorcluster)
            n89 = case shown="False" FALSE {
              tunnel: w265 -> [w273 _]
              tunnel: [w273 _] -> w264
              frame False {
              }
              frame True {
              }
            }
            n90 = case shown="True" w262 {
              tunnel: w261 -> [w270 w272]
              tunnel: [w270 w271] -> w258
              frame False {
                # "These are the remaining states (at the moment the error occured). States can be altered according to business logic."
                # "NOT SHUTTING DOWN"
              }
              frame True {
                # "Developer can decide to alter the states but should be aware that during the shutdown process, there are certain states that must be run for the SMO to properly shut itself (and this process) down. As such, one can add states to perform additional clean-ups, but should append the remaining state to be executed."
                # "SHUTTING DOWN"
                n91 = call <vilib>:"Add State(s) to Queue__jki_lib_state_machine.vi"("State(s) in (\"\")"=w272) -> ("States Out"=w271:string)  [unwired: 14 in]
              }
            }
            n92 = Bundle By Name(cluster=w259, "Core.Last Error.error"=w264) -> (w260:T6)
            n93 = call <vilib>:"Add State(s) to Queue__jki_lib_state_machine.vi"("State(s) in Front (\"\")"=w258, "State(s) in (\"\")"=w269) -> ("States Out"=w268:string)  [unwired: 13 in]
          }
          frame "Macro: Run Sequence" {
            # "0,1,2,3,4,"
            # "5"
            # "Do not put any code in this frame.\n(It is a separator no-op. You can make a copy of this frame to create a new Macro frame)"
            n94 = Unbundle By Name(w280) -> ("sequence"=w276:string[], "Running Step"=w274:i32)
            n95 = Array Size(array=w276) -> (size(s)=w286:i32)
            n96 = Index Array(array=w276, index=w274) -> (element=w275:string)
            n97 = Greater Or Equal?(x=w286, y=w274) -> (x >= y?=w278:bool)
            n98 = Select(t=-1 ("Running Step"), s=w278, f=w274) -> (s? t:f=w285:i32)
            n99 = Bundle By Name(cluster=w280, "Running Step"=w285) -> (w281:T6)
            n100 = Select(t="Sequence: Status >> ...", s=w278, f="Idle //Check Event Structure\nMacro: Run Sequence" ("State(s) at Back (\"\")")) -> (s? t:f=w277:string)
            n101 = call <vilib>:"Add State(s) to Queue__jki_lib_state_machine.vi"("State(s) in Front (\"\")"=w275, "State(s) at Back (\"\")"=w277) -> ("States Out"=w279:string)  [unwired: 13 in]
            n102 = call <vilib>:"Add State(s) to Queue__jki_lib_state_machine.vi"("State(s) in Front (\"\")"=w279, "State(s) in (\"\")"=w290) -> ("States Out"=w289:string)  [unwired: 13 in]
          }
          frame "Macro: Exit" {
            # "Exit Macro\n(This is called once, when the VI exits)"
            n103 = Unbundle By Name(w291) -> ("Core.Close Panel on Exit?"=w305:bool)
            n104 = Bundle By Name(cluster=w291, "Core.Shutdown?"=TRUE) -> (w292:T6)
            n105 = Select(t="UI: Front Panel State >> Close", s=w305, f="" ("Empty String Constant")) -> (s? t:f=w303:string)
            n106 = call <vilib>:"Add State(s) to Queue__jki_lib_state_machine.vi"("State(s) in Front (\"\")"="Data: Cleanup\nEvents: Unregister", "State(s) in (\"\")"="Process: Sync", "State(s) at Back (\"\")"="Exit") -> ("States Out"=w298:string)  [unwired: 12 in]
            n107 = call <vilib>:"Add State(s) to Queue__jki_lib_state_machine.vi"("State(s) in Front (\"\")"="Instrument: Close Hardware", "State(s) in (\"\")"=w303, "State(s) at Back (\"\")"=w298) -> ("States Out"=w302:string)  [unwired: 12 in]
            n108 = call <vilib>:"Add State(s) to Queue__jki_lib_state_machine.vi"("State(s) in Front (\"\")"=w302, "State(s) in (\"\")"=w307) -> ("States Out"=w306:string)  [unwired: 13 in]
          }
          frame "---------- Process ----------" {
            # "Template Separator\n(You can make a copy of, or modify, this frame)"
            n109 = call <vilib>:"Add State(s) to Queue__jki_lib_state_machine.vi"("State(s) in (\"\")"=w312) -> ("States Out"=w311:string)  [unwired: 14 in]
          }
          frame "Process: Sync" {
            n110 = Unbundle By Name(w320) -> ("SelfRef"=w316:refnum<class "Inst.RP100.lvclass">)
            n111 = call <vilib>:"WaitOnProcessSync.vi"("error in (no error)"=w315, "SMO"=w316) -> ("error out"=w314:errorcluster, "Don't run?"=w319:bool)  [unwired: 7 in, 1 out]
            n112 = Select(t="Data: Cleanup\nEvents: Unregister\nExit", s=w319, f="" ("Empty String Constant")) -> (s? t:f=w313:string)
            n113 = call <vilib>:"Add State(s) to Queue__jki_lib_state_machine.vi"("State(s) in Front (\"\")"=w313, "State(s) in (\"\")"=w323) -> ("States Out"=w322:string)  [unwired: 13 in]
          }
          frame "---------- Events ----------" {
            # "Template Separator\n(You can make a copy of, or modify, this frame)"
            n114 = call <vilib>:"Add State(s) to Queue__jki_lib_state_machine.vi"("State(s) in (\"\")"=w328) -> ("States Out"=w327:string)  [unwired: 14 in]
          }
          frame "Events: Register" {
            n115 = Unbundle By Name(w334) -> ("SelfRef"=w335:refnum<class "Inst.RP100.lvclass">)
            n116 = call <vilib>:"GetProtectedEvents.vi"("SMO"=w335) -> ("error out"=w333:errorcluster, "SMO Protected Events"=w338:T9, "SMO out"=w332:refnum<class "Inst.RP100.lvclass">)  [unwired: 8 in]
            n117 = call "Inst.RP100.GetPrivateEvents.vi"("Inst.RP100 in"=w332) -> ("error out"=w329:errorcluster, "Inst.RP100 Private Events"=w330:cluster{"MessageToProcess":refnum<user-event>})  [unwired: 8 in, 1 out]
            n118 = register-events(w338, w330) -> (reference out=w339:refnum<event-registration>, error out=w336:errorcluster)  [unwired: 2 in]
            n119 = Merge Errors(w336, w329, w333, w331) -> (w337:errorcluster)
            n120 = call <vilib>:"Add State(s) to Queue__jki_lib_state_machine.vi"("State(s) in (\"\")"=w341) -> ("States Out"=w340:string)  [unwired: 14 in]
          }
          frame "Events: Unregister" {
            n121 = Unregister For Events(event registration refnum=w344, error in=w343) -> (error out=w342:errorcluster)
            n122 = call <vilib>:"Clear Errors.vi"("error in (no error)"=w342) -> ()  [unwired: 5 in, 2 out]
            n123 = call <vilib>:"Add State(s) to Queue__jki_lib_state_machine.vi"("State(s) in (\"\")"=w347) -> ("States Out"=w346:string)  [unwired: 14 in]
          }
          frame "---------- Instrument ----------" {
            n124 = Unbundle By Name(w349) -> ("SelfRef"=w348:refnum<class "Inst.RP100.lvclass">)
            n125 = Bundle By Name(cluster=w349, "SelfRef"=w348) -> (w350:T6)
            n126 = call <vilib>:"Add State(s) to Queue__jki_lib_state_machine.vi"("State(s) in (\"\")"=w354) -> ("States Out"=w353:string)  [unwired: 14 in]
          }
          frame "Instrument: Open Hardware" {
            n127 = Unbundle By Name(w359) -> ("SelfRef"=w358:refnum<class "Inst.RP100.lvclass">)
            n128 = call-dynamic "Open Hardware.vi"("error in (no error)"=w355, "Inst.RP100 in"=w358) -> ("error out"=w356:errorcluster, "Inst.RP100 out"=w357:refnum<class "Inst.RP100.lvclass">)  [unwired: 8 in]
            n129 = Bundle By Name(cluster=w359, "SelfRef"=w357) -> (w360:T6)
            n130 = call <vilib>:"Add State(s) to Queue__jki_lib_state_machine.vi"("State(s) in (\"\")"=w363) -> ("States Out"=w362:string)  [unwired: 14 in]
          }
          frame "Instrument: Close Hardware" {
            n131 = Unbundle By Name(w368) -> ("SelfRef"=w367:refnum<class "Inst.RP100.lvclass">)
            n132 = call-dynamic "Close Hardware.vi"("error in (no error)"=w364, "Inst.RP100 in"=w367) -> ("error out"=w365:errorcluster, "Inst.RP100 out"=w366:refnum<class "Inst.RP100.lvclass">)  [unwired: 8 in]
            n133 = Bundle By Name(cluster=w368, "SelfRef"=w366) -> (w369:T6)
            n134 = call <vilib>:"Add State(s) to Queue__jki_lib_state_machine.vi"("State(s) in (\"\")"=w372) -> ("States Out"=w371:string)  [unwired: 14 in]
          }
          frame "Instrument: setLevel" {
            # "communicate with\nhardware"
            n135 = Unbundle By Name(w378) -> ("SelfRef"=w376:refnum<class "Inst.RP100.lvclass">, "MessageToProcess.Message.Data"=w373:variant)  [unwired: 1 out]
            n136 = call "Inst.RP100.setLevel.vi"("error in (no error)"=w375, "Variant"=w373, "Inst.RP100 out"=w376) -> ("error out"=w374:errorcluster, "Inst.RP100 out"=w377:refnum<class "Inst.RP100.lvclass">)  [unwired: 7 in]
            n137 = Bundle By Name(cluster=w378, "SelfRef"=w377) -> (w379:T6)
            n138 = call <vilib>:"Add State(s) to Queue__jki_lib_state_machine.vi"("State(s) in (\"\")"=w382) -> ("States Out"=w381:string)  [unwired: 14 in]
          }
          frame "Instrument: setStrain" {
            # "communicate with\nhardware"
            n139 = Unbundle By Name(w388) -> ("SelfRef"=w386:refnum<class "Inst.RP100.lvclass">, "MessageToProcess.Message.Data"=w383:variant)  [unwired: 1 out]
            n140 = call "Inst.RP100.setStrain.vi"("error in (no error)"=w385, "data in"=w383, "Inst.RP100 in"=w386) -> ("error out"=w384:errorcluster, "Inst.RP100 out"=w387:refnum<class "Inst.RP100.lvclass">)  [unwired: 7 in]
            n141 = Bundle By Name(cluster=w388, "SelfRef"=w387) -> (w389:T6)
            n142 = call <vilib>:"Add State(s) to Queue__jki_lib_state_machine.vi"("State(s) in (\"\")"=w392) -> ("States Out"=w391:string)  [unwired: 14 in]
          }
          frame "Instrument: setState" {
            # "communicate with\nhardware"
            n143 = Unbundle By Name(w398) -> ("SelfRef"=w396:refnum<class "Inst.RP100.lvclass">, "MessageToProcess.Message.Data"=w393:variant)  [unwired: 1 out]
            n144 = call "Inst.RP100.setState.vi"("error in (no error)"=w395, "data in"=w393, "Inst.RP100 in"=w396) -> ("error out"=w394:errorcluster, "Inst.RP100 out"=w397:refnum<class "Inst.RP100.lvclass">)  [unwired: 7 in]
            n145 = Bundle By Name(cluster=w398, "SelfRef"=w397) -> (w399:T6)
            n146 = call <vilib>:"Add State(s) to Queue__jki_lib_state_machine.vi"("State(s) in (\"\")"=w402) -> ("States Out"=w401:string)  [unwired: 14 in]
          }
          frame "Instrument: getAll" {
            # "communicate with\nhardware"
            n147 = Unbundle By Name(w410) -> ("SelfRef"=w409:refnum<class "Inst.RP100.lvclass">)  [unwired: 2 out]
            n148 = call "Inst.RP100.getAll.vi"("error in (no error)"=w408, "Inst.RP100 in"=w409) -> ("error out"=w404:errorcluster, "output cluster"=w407:T10, "Inst.RP100 out"=w406:refnum<class "Inst.RP100.lvclass">)  [unwired: 7 in]
            n149 = call <userlib>:"setAllData.vi"("error in (no error)"=w404, "AllData"=w407, "Instrument in"=w406) -> ("error out"=w403:errorcluster, "Instrument out"=w405:refnum<class "Inst.RP100.lvclass">)  [unwired: 7 in]
            n150 = Bundle By Name(cluster=w410, "SelfRef"=w405) -> (w411:T6)
            n151 = call <vilib>:"Add State(s) to Queue__jki_lib_state_machine.vi"("State(s) in (\"\")"=w414) -> ("States Out"=w413:string)  [unwired: 14 in]
          }
          frame "Instrument: Log" {
            n152 = Unbundle By Name(w423) -> ("SelfRef"=w416:refnum<class "Inst.RP100.lvclass">)
            n153 = Unbundle By Name(w416) -> ("Data"=w420:T10)
            n154 = call-dynamic "Get SMO PGSQL Log Paths.vi"("error in (no error)"=w418, "Inst.RP100 in"=w416) -> ("error out"=w419:errorcluster, "Paths"=w422:string, "Inst.RP100 out"=w421:refnum<class "Inst.RP100.lvclass">)  [unwired: 7 in]
            n155 = call <userlib>:"Instrument.logToDatabase.vi"("error in (no error)"=w419, "Data"=w420, "Paths"=w422, "Instrument"=w421) -> ("error out"=w417:errorcluster, "Instrument out"=w415:refnum<class "Inst.RP100.lvclass">)  [unwired: 6 in]
            n156 = Bundle By Name(cluster=w423, "SelfRef"=w415) -> (w424:T6)
            n157 = call <vilib>:"Add State(s) to Queue__jki_lib_state_machine.vi"("State(s) in (\"\")"=w427) -> ("States Out"=w426:string)  [unwired: 14 in]
          }
          frame "---------- Sequence ----------" {
            n158 = call <vilib>:"Add State(s) to Queue__jki_lib_state_machine.vi"("State(s) in (\"\")"=w432) -> ("States Out"=w431:string)  [unwired: 14 in]
          }
          frame "Sequence: Status" {
            # "Sequence: Status\n(Use this frame to pass the status to the UI, this VI's UI, etc)"
            n159 = call <vilib>:"Add State(s) to Queue__jki_lib_state_machine.vi"("State(s) in (\"\")"=w438) -> ("States Out"=w437:string)  [unwired: 14 in]
            "Status" <- w433
          }
          frame "Sequence: Wait" {
            # "Sequence: Wait\n(Non-Blocking Wait)"
            # "F = repeat this state. wait\nT = go to next state. don't wait"
            n160 = Unbundle By Name(w447) -> ("Running Step"=w440:i32)
            n161 = call <userlib>:"Wait Logic.vi"("error in (no error)"=w443, "Time"=w441) -> ("error out"=w442:errorcluster, "Status String"=w439:string, "Trigger"=w444:bool)  [unwired: 6 in, 1 out]
            n162 = Increment(x=w440) -> (x+1=w454:i32)
            n163 = Select(t=w454, s=w444, f=w440) -> (s? t:f=w445:i32)
            n164 = Select(t=u32 0, s=w444, f=u32 100 ("milliseconds to wait")) -> (s? t:f=w451:u32)
            n165 = call <userlib>:"Wait (ms)__ogtk.vi"("error in (no error)"=w442, "milliseconds to wait"=w451) -> ("error out"=w449:errorcluster)  [unwired: 8 in, 1 out]
            n166 = Bundle By Name(cluster=w447, "Running Step"=w445) -> (w446:T6)
            n167 = call <vilib>:"Build State String with Arguments__JKI_lib_State_Machine.vi"("Arguments (\"\")"=w439, "State"="Sequence: Status") -> ("State with Arguments"=w448:string)  [unwired: 4 in]
            n168 = call <vilib>:"Add State(s) to Queue__jki_lib_state_machine.vi"("State(s) in Front (\"\")"=w448, "State(s) in (\"\")"=w457) -> ("States Out"=w456:string)  [unwired: 13 in]
          }
        }
      }
    }
    frame Error {
    }
  }
  n169 = call-parent "Process.vi"("error in"=w5, "Instrument"=w4) -> ("error out"=w2:errorcluster, "Instrument out"=→"Inst.RP100 out":refnum<class "Inst.RP100.lvclass">)  [unwired: 8 in]
  n170 = Merge Errors(w2, w1) -> (→"error out":errorcluster)
